vi "CheckUsernamePassword.vi"(8 "error in (no error)":errorcluster, 9 "Password":string, 10 "Username":string, 11 "Array":string[][](array[string])) -> (0 "error out":errorcluster, 1 "Index of user":i32, 3 "User exists":bool)   [LabVIEW 2017]
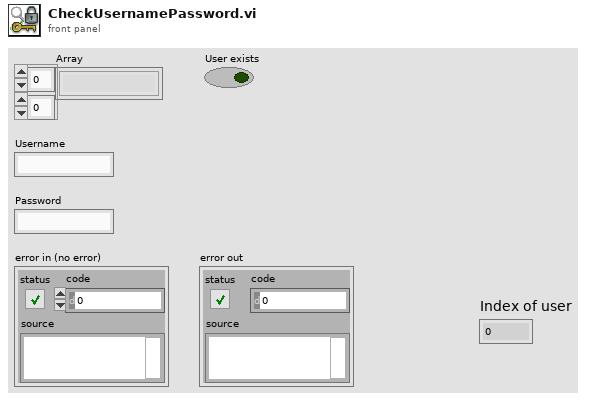
[diagram p1: front panel]
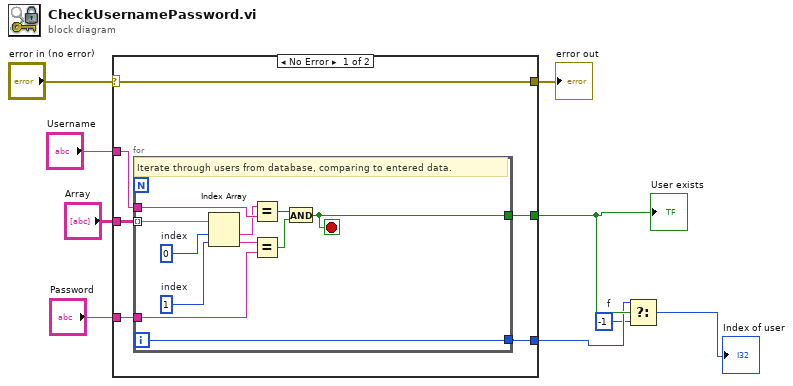
[diagram p0: block diagram]
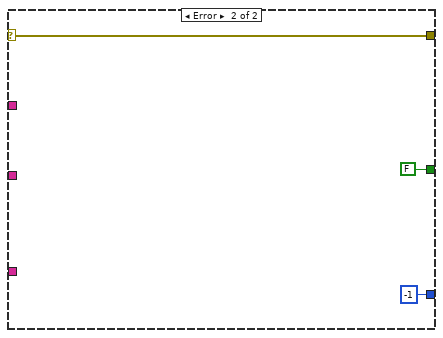
[diagram p2: hidden frame]
diagram:
  w2 = -1  # f
  n1 = case shown="No Error" "error in (no error)" {
    selector: "error in (no error)" -> [w11 w29]
    tunnel: [w15 FALSE] -> w4
    tunnel: "Array" -> [w14 _]
    tunnel: "Password" -> [w13 _]
    tunnel: "Username" -> [w12 _]
    tunnel: [w11 w29] -> w5
    tunnel: [w10 -1] -> w3
    frame No Error {
      n2 = for {
        tunnel: w12 -> [w24]
        tunnel: w13 -> [w23]
        tunnel: [w20] -> w15
        tunnel: w14 -> [w19] mode=indexing
        tunnel: [w16] -> w10
        i -> [w16]
        stop <- w20 stop-if-true
        w25 = 1  # index
        w26 = 0  # index
        # "Iterate through users from database, comparing to entered data."
        n3 = Index Array(array=w19, index #1=w26, index #2=w25) -> (element #1=w18:string, element #2=w17:string)
        n4 = Equal?(x=w18, y=w24) -> (x = y?=w22:bool)
        n5 = Equal?(x=w17, y=w23) -> (x = y?=w21:bool)
        n6 = And(x=w22, y=w21) -> (x .and. y?=w20:bool)
      }
    }
    frame Error {
    }
  }
  "error out" <- w5
  "User exists" <- w4
  n7 = Select(t=w3, s=w4, f=w2) -> (s? t:f=→"Index of user":i32)
